vi "Advantech TC Example.vi"() -> ()   [LabVIEW 2019]
uses:
  <userlib>/DAQNavi Polymorphic VI/configure/DAQNavi Get Property/Device/DAQNaviGet_Device_SupportedDevices.vi
  <userlib>/DAQNavi Polymorphic VI/create/DAQNavi Create Channel(AI-Temperature).vi
  <userlib>/DAQNavi Polymorphic VI/read/DAQNavi Read (Analog 1D DBL NChan 1Samp).vi
panel:
  in  "Scan Rate (mS)":u32=500
  out "Temperature Response":T1(graph)
  in  "stop":bool
  out "Temperature 3 (°F)":dbl format="%#.2g"
  out "Temperature 2 (°F)":dbl format="%#.2g"
  out "Temperature 1 (°F)":dbl format="%#.2g"
  out "error out":errorcluster
  out "task out":i32
  in  "error in (no error)":errorcluster
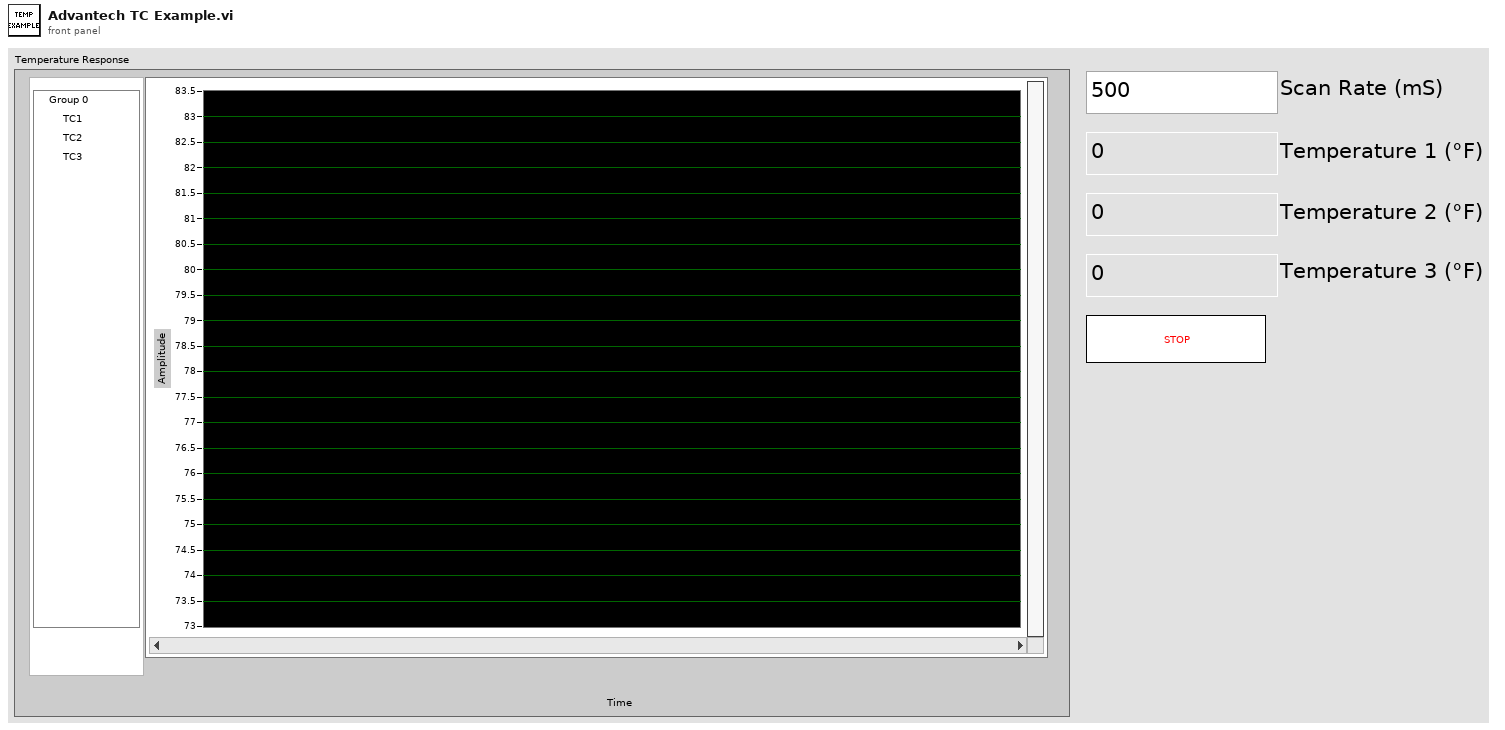
[diagram p1: front panel]
types:
  T1 = cluster{"Waveform Graph":waveform(dbl), "Waveform Graph":waveform(dbl), "Waveform Graph":waveform(dbl)}
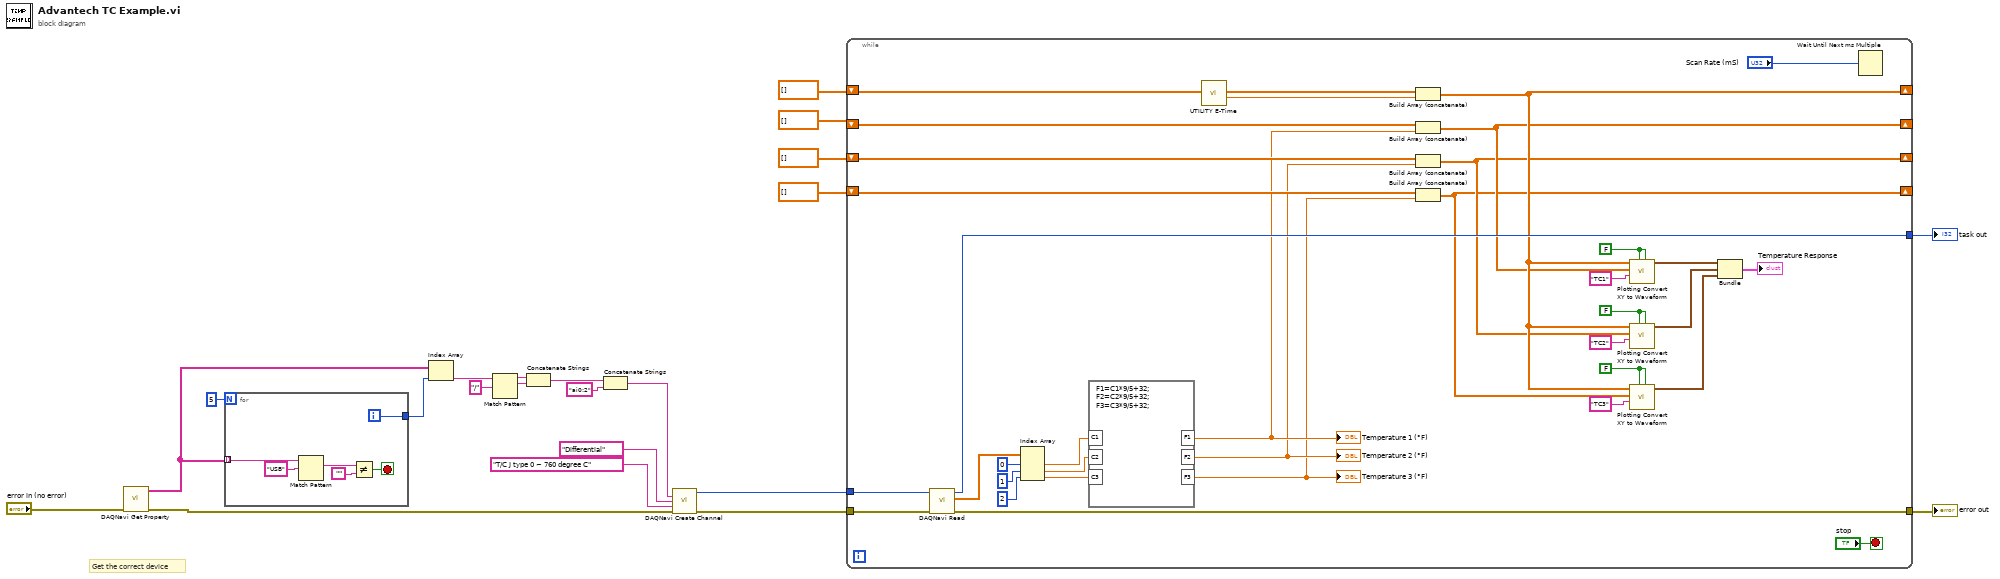
[diagram p0: block diagram]
diagram:
  # "Get the correct device"
  n1 = call-poly <userlib>:"DAQNavi Get Property.vi"("error in (no error)"="error in (no error)") -> ("error out"=w10:errorcluster, "supported devices"=w20:string[])  [unwired: 9 in]
  n2 = for {
    N: 5 -> [_]
    tunnel: w20 -> [w28] mode=indexing
    tunnel: [w26] -> w22
    i -> [w26]
    stop <- w24 stop-if-true
    n3 = Match Pattern(string=w28, regular expression="USB") -> (match substring=w23:string)  [unwired: 1 in, 3 out]
    n4 = Not Equal?(x=w23, y="") -> (x != y?=w24:bool)
  }
  n5 = Index Array(array=w20, index=w22) -> (element=w14:string)
  n6 = Match Pattern(string=w14, regular expression="/") -> (before substring=w16:string, match substring=w17:string)  [unwired: 1 in, 2 out]
  n7 = Concatenate Strings(w16, w17) -> (w19:string)
  n8 = Concatenate Strings(w19, "ai0:2") -> (w9:string)
  n9 = call-poly <userlib>:"DAQNavi Create Channel.vi"("physical channels"=w9, "signal type"="Differential", "value range"="T/C J type 0 ~ 760 degree C", "error in (no error)"=w10) -> ("task out"=w8:i32, "error out"=w7:errorcluster)  [unwired: 10 in]
  n10 = while {
    tunnel: w8 -> [w63]
    tunnel: w7 -> [w62]
    tunnel: [w53] -> w6
    tunnel: [w52] -> w5
    shift-right: [w46] -> _
    shift-left: dbl[] [] -> [w50]
    shift-right: [w45] -> _
    shift-left: dbl[] [] -> [w49]
    shift-right: [w44] -> _
    shift-left: dbl[] [] -> [w48]
    shift-right: [w43] -> _
    shift-left: dbl[] [] -> [w47]
    stop <- "stop" stop-if-true
    w29 = FALSE ("Use Filter?")
    w30 = FALSE ("Use Filter?")
    w31 = FALSE ("Use Filter?")
    n11 = call-poly <userlib>:"DAQNavi Read.vi"("error in (no error)"=w62, "task in"=w63) -> ("error out"=w53:errorcluster, "data"=w58:dbl[], "task out"=w52:i32)  [unwired: 7 in]
    n12 = Index Array(array=w58, index #1=0 ("index"), index #2=1 ("index"), index #3=2 ("index")) -> (element #1=w57:dbl, element #2=w56:dbl, element #3=w55:dbl)
    n13 = formula code="F1=C1*9/5+32;\nF2=C2*9/5+32;\nF3=C3*9/5+32;"("C1"=w57, "C2"=w56, "C3"=w55) -> ("F1"=w35:dbl, "F2"=w34:dbl, "F3"=w33:dbl)
    "Temperature 1 (°F)" <- w35
    "Temperature 2 (°F)" <- w34
    "Temperature 3 (°F)" <- w33
    n14 = call "UTILITY E-Time.vi"() -> ("Elapsed Time (sec)"=w32:dbl)  [unwired: 9 in, 2 out]
    n15 = Build Array (concatenate)(w50, w32) -> (w46:dbl[])
    n16 = Build Array (concatenate)(w49, w35) -> (w45:dbl[])
    n17 = Build Array (concatenate)(w48, w34) -> (w44:dbl[])
    n18 = Build Array (concatenate)(w47, w33) -> (w43:dbl[])
    n19 = call "Plotting Convert XY to Waveform.vi"("Macro Filter"=w31, "Use Filter?"=w31, "Plot Name"="TC1", "Y"=w45, "X"=w46) -> ("Waveform Graph"=w42:waveform(dbl))  [unwired: 4 in, 2 out]
    n20 = call "Plotting Convert XY to Waveform.vi"("Macro Filter"=w30, "Use Filter?"=w30, "Plot Name"="TC2", "Y"=w44, "X"=w46) -> ("Waveform Graph"=w41:waveform(dbl))  [unwired: 4 in, 2 out]
    n21 = call "Plotting Convert XY to Waveform.vi"("Macro Filter"=w29, "Use Filter?"=w29, "Plot Name"="TC3", "Y"=w43, "X"=w46) -> ("Waveform Graph"=w40:waveform(dbl))  [unwired: 4 in, 2 out]
    n22 = Bundle "Bundle"("Waveform Graph"=w42, "Waveform Graph"=w41, "Waveform Graph"=w40) -> (→"Temperature Response":T1)  [unwired: 1 in]
    n23 = Wait Until Next ms Multiple(millisecond multiple="Scan Rate (mS)") -> ()  [unwired: 1 out]
  }
  "error out" <- w6
  "task out" <- w5
